vi "Main.vi"(11 "Module Admin":refnum<class "Delacor_lib_QMH_Module Admin.lvclass">) -> ()   [LabVIEW 2024, in "UI Module Template.lvlib"]
doc: "This template is based off of the Queued Message Handler design pattern and the Queued Message Handler project template that ships with LabVIEW.\n\nThe main difference is that the queue is private to this module and communication between modules is performed via Broadcast and Request events.\n\nRequest events are wrapped in public API methods and are handled in the Event Handling Loop (EHL) of this VI. Any module can register for Broadcast events sent by this module. The EHL generates messages based on user interface actions.\n\nThe Message Handling Loop (MHL) processes messages generated by the EHL, or by other messages. The messages are string values, so new messages can be added easily to the Message Cases case structure in the MHL. Each message cluster can also provide an optional value for Message Data, which is a variant that can be converted to whatever message-specific data is required.\n_____\nBased on DQMH Project Template 7.0.1.1316."
uses:
  UI Module Template.lvlib
  <vilib>/Delacor/Delacor QMH/Libraries/Module Admin_class/Delacor_lib_QMH_Module Admin.lvclass
  Module Data--cluster.ctl
  Config.ctl
  <vilib>/Delacor/Delacor QMH/Libraries/Message Queue_class/Delacor_lib_QMH_Message Queue.lvclass/Delacor_lib_QMH_Message Queue.ctl
  Stop Argument--cluster.ctl
  <vilib>/Delacor/Delacor QMH/Libraries/Module Admin_class/Delacor_lib_QMH_Module Admin.lvclass/Delacor_lib_QMH_Module Admin.ctl
  Get UI Reference Argument--cluster.ctl
  Get UI Reference (Reply Payload)--cluster.ctl
  Inserted Into Subpanel Argument--cluster.ctl
  Set Config (String) Argument--cluster.ctl
  Set Config Argument--cluster.ctl
  Get config Argument--cluster.ctl
  Get config (Reply Payload)--cluster.ctl
  Get Config (String) Argument--cluster.ctl
  Get Config (String) (Reply Payload)--cluster.ctl
  Generate Dummy Data Argument--cluster.ctl
  <vilib>/Delacor/Delacor QMH/Libraries/Message Queue_class/Delacor_lib_QMH_Enqueue Message (Single).vi
  <vilib>/Delacor/Delacor QMH/Libraries/Module Admin_class/Delacor_lib_QMH_Get External Launch.vi
  <vilib>/Delacor/Delacor QMH/Libraries/Message Queue_class/Delacor_lib_QMH_Message Queue.lvclass
  <userlib>/_OpenG.lib/appcontrol/appcontrol.llb/openg_application_control.lvlib
panel:
  out "Title":string
  out "error out":errorcluster
  out "Status":string
  in  "Simulate MHL Error":bool
  in  "Simulate EHL Error":bool
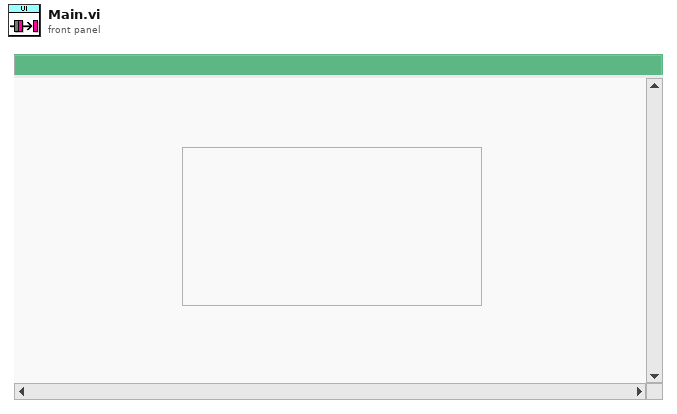
[diagram p1: front panel]
types:
  T1 = typedef "UI Module Template.lvlib/Request Events--cluster.ctl" = cluster{"Stop Module":refnum<user-event>, "Show Panel":refnum<user-event>, "Hide Panel":refnum<user-event>, "Get Module Execution Status":refnum<user-event>, "Show Diagram":refnum<user-event>, "Get UI Reference":refnum<user-event>, "Inserted Into Subpanel":refnum<user-event>, "Set Config (String)":refnum<user-event>, "Set Config":refnum<user-event>, "Get config":refnum<user-event>, "Get Config (String)":refnum<user-event>, "Private":cluster{"Generate Dummy Data":refnum<user-event>}}
  T2 = typedef "UI Module Template.lvlib/Module Data--cluster.ctl" = cluster{"Status":string, "Config":T3}
  T3 = typedef "UI Module Template.lvlib/Config.ctl" = cluster{"<ReplaceMe>":bool}
  T4 = enum32{"invalid lock state", "Not Locked", "Locked (No Password)", "Password-protected"}
  T5 = typedef "UI Module Template.lvlib/Stop Argument--cluster.ctl" = cluster{"Origin":string, "Exit via Stop Module Req?":bool, "Wait for Module to stop?":bool}
  T6 = typedef "UI Module Template.lvlib/Get UI Reference Argument--cluster.ctl" = cluster{"Wait Notifier":refnum<notifier>, "wait for reply":bool}
  T7 = typedef "UI Module Template.lvlib/Inserted Into Subpanel Argument--cluster.ctl" = cluster{"Boolean":bool}
  T8 = typedef "UI Module Template.lvlib/Set Config (String) Argument--cluster.ctl" = cluster{"XML-String":string}
  T9 = typedef "UI Module Template.lvlib/Set Config Argument--cluster.ctl" = cluster{"Config":T3}
  T10 = typedef "UI Module Template.lvlib/Get config Argument--cluster.ctl" = cluster{"Wait Notifier":refnum<notifier>, "wait for reply":bool}
  T11 = typedef "UI Module Template.lvlib/Get Config (String) Argument--cluster.ctl" = cluster{"Wait Notifier":refnum<notifier>, "wait for reply":bool}
  T12 = typedef "UI Module Template.lvlib/Generate Dummy Data Argument--cluster.ctl" = cluster{"Boolean":bool}
  T13 = enum32{"Invalid", "Standard", "Closed", "Hidden", "Minimized", "Maximized"}
  T14 = typedef "UI Module Template.lvlib/Get UI Reference (Reply Payload)--cluster.ctl" = cluster{"UI VI Refnum":refnum<vi>, "error":errorcluster}
  T15 = typedef "UI Module Template.lvlib/Get config (Reply Payload)--cluster.ctl" = cluster{"Config":T3, "error":errorcluster}
  T16 = typedef "UI Module Template.lvlib/Get Config (String) (Reply Payload)--cluster.ctl" = cluster{"Config XML String":string, "error":errorcluster}
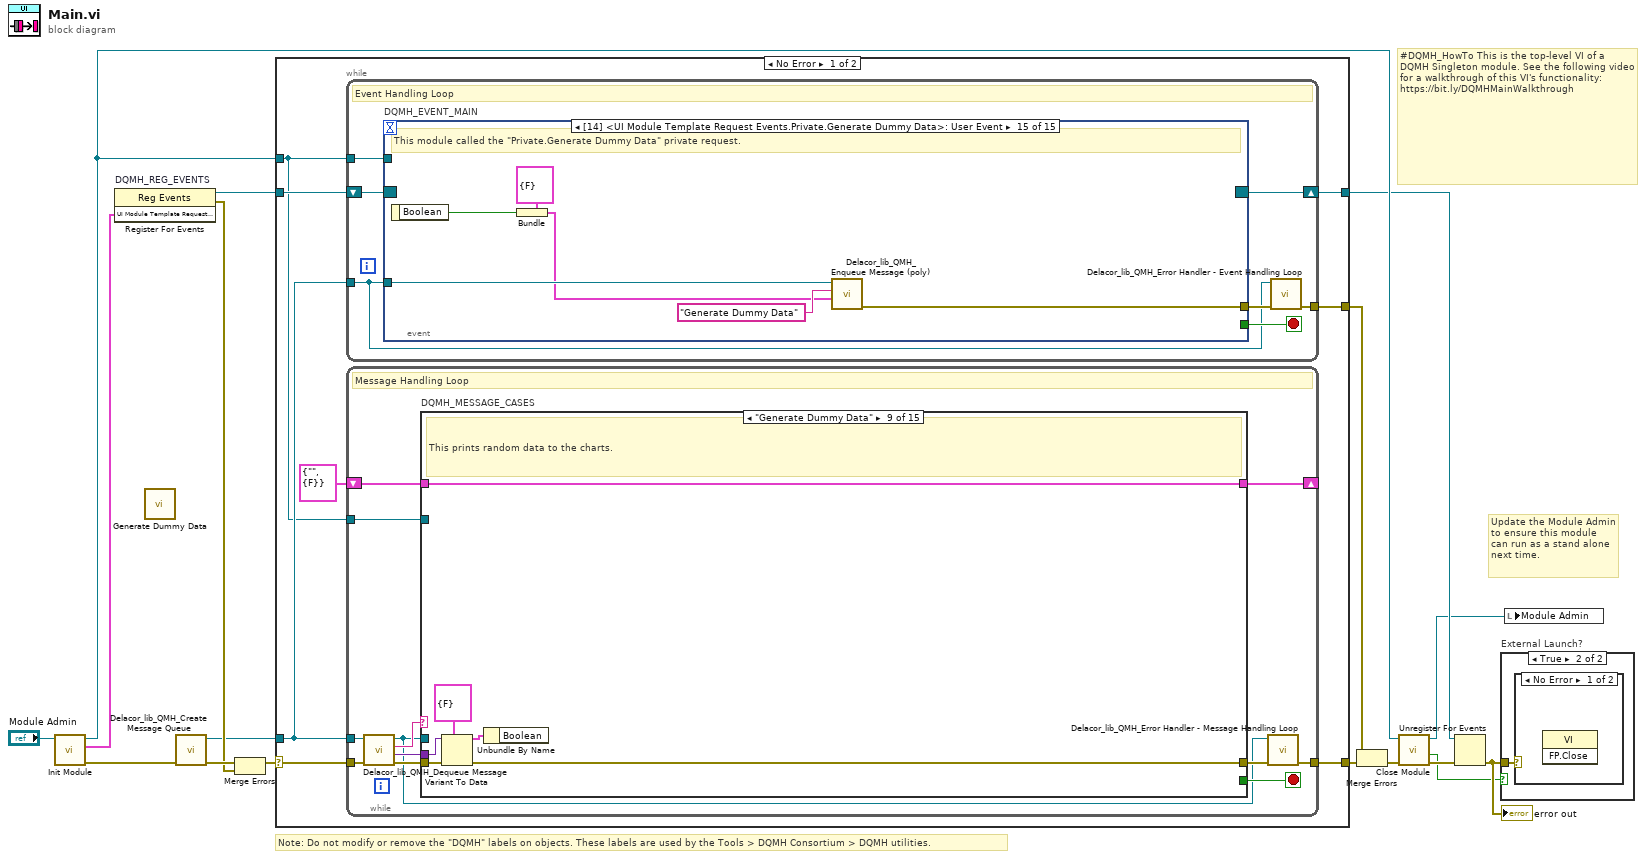
[diagram p0: block diagram]
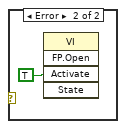
[diagram p3: hidden frame]
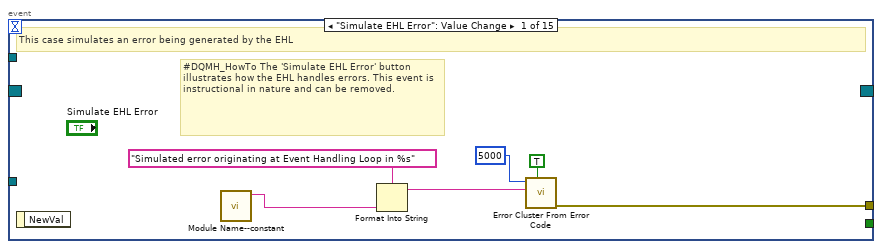
[diagram p4: hidden frame]
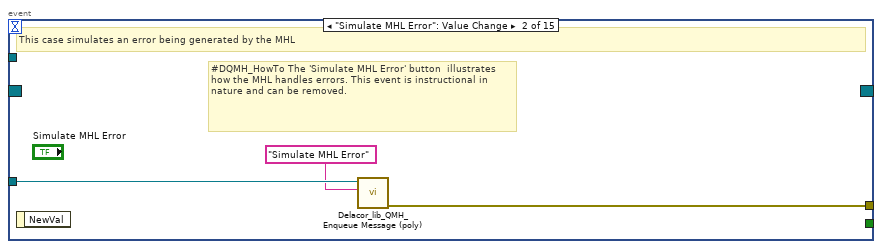
[diagram p5: hidden frame]
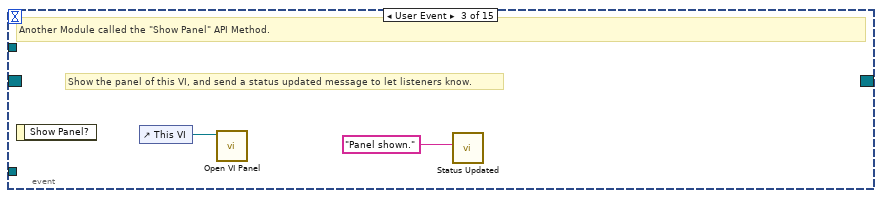
[diagram p6: hidden frame]
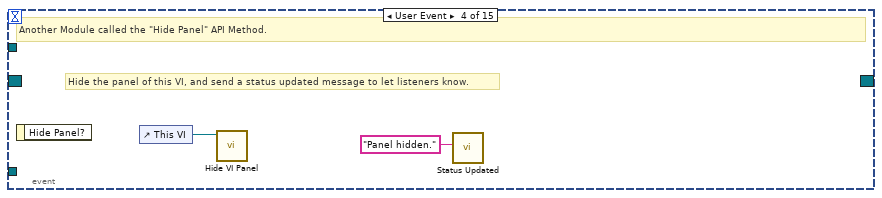
[diagram p7: hidden frame]
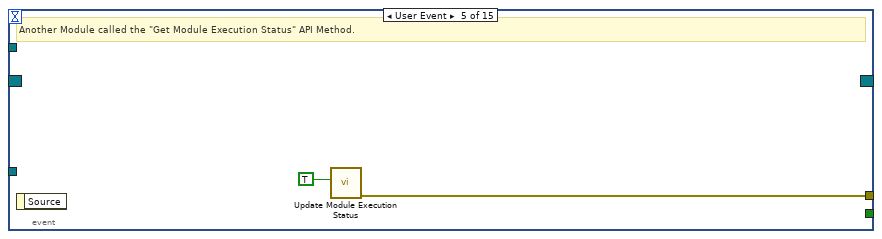
[diagram p8: hidden frame]
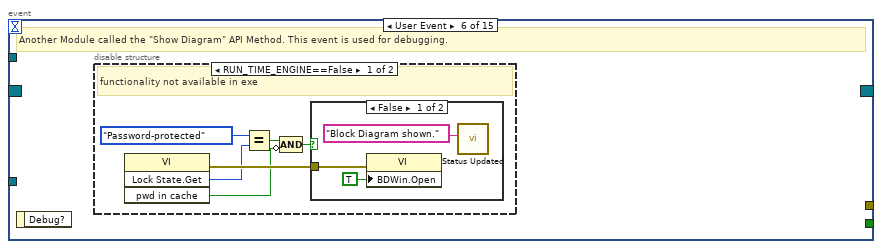
[diagram p9: hidden frame]
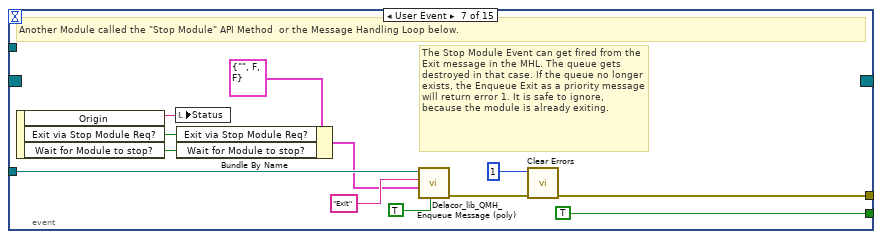
[diagram p12: hidden frame]
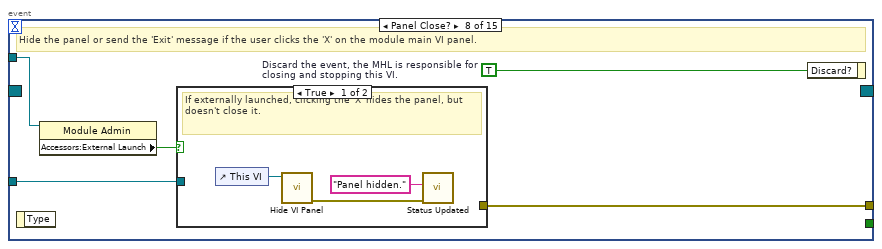
[diagram p13: hidden frame]
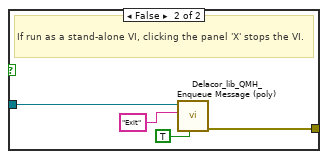
[diagram p14: hidden frame]
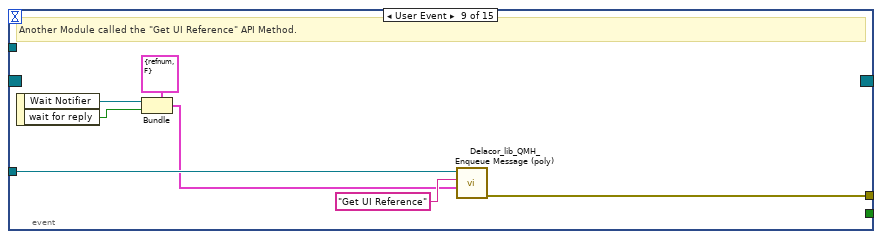
[diagram p15: hidden frame]
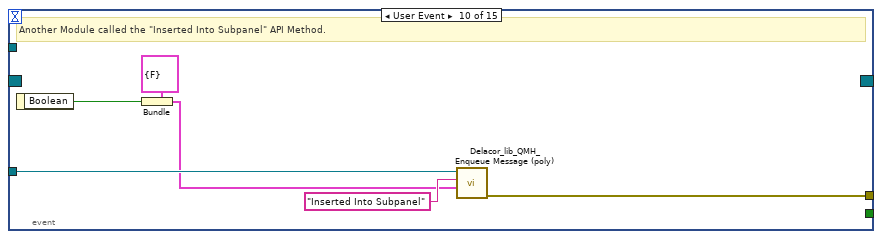
[diagram p16: hidden frame]
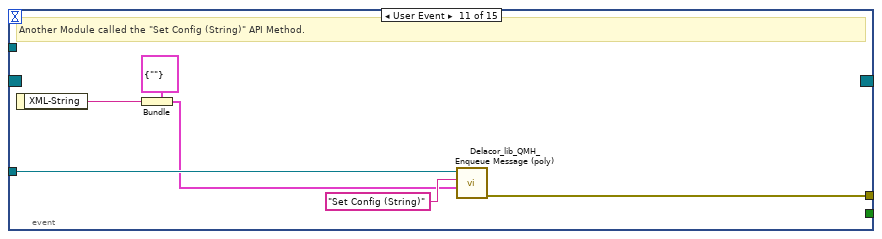
[diagram p17: hidden frame]
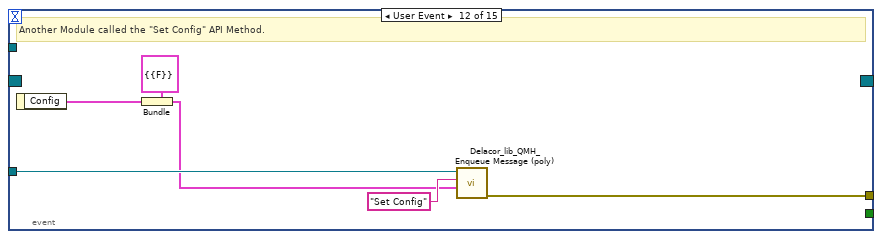
[diagram p18: hidden frame]
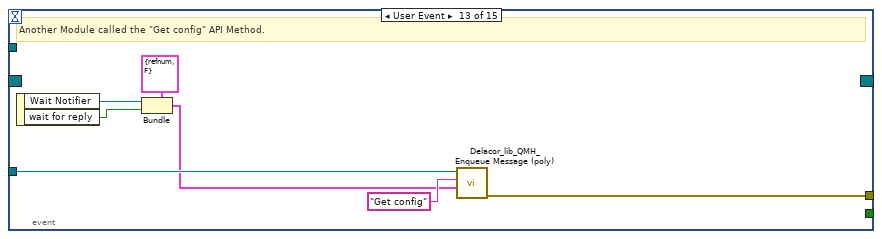
[diagram p19: hidden frame]
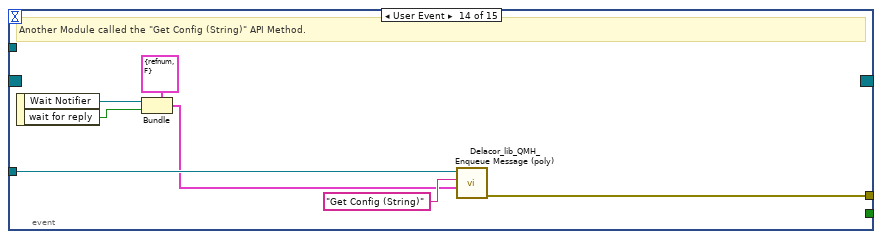
[diagram p20: hidden frame]
diagram:
  # "#DQMH_HowTo This is the top-level VI of a DQMH Singleton module. See the following video for a walkthrough of this VI's functionality: https://bit.ly/DQMHMainWalkthrough"
  # "Note: Do not modify or remove the \"DQMH\" labels on objects. These labels are used by the Tools > DQMH Consortium > DQMH utilities."
  # "Update the Module Admin to ensure this module can run as a stand alone next time."
  n1 = call "Init Module.vi"("Singleton Module Admin in"="Module Admin") -> ("error out"=w16:errorcluster, "UI Module Template Request Events"=w5:T1, "Singleton Module Admin out"=w8:refnum<class "Delacor_lib_QMH_Module Admin.lvclass">)  [unwired: 8 in]
  n2 = register-events "DQMH_REG_EVENTS"(w5) -> (reference out=w6:refnum<event-registration>, error out=w9:errorcluster)  [unwired: 2 in]
  n3 = call "Generate Dummy Data.vi"() -> ()  [unwired: 11 in, 1 out]
  n4 = call <vilib>:"Delacor_lib_QMH_Create Message Queue.vi"("error in"=w16) -> ("error out"=w11:errorcluster, "Message Queue"=w4:refnum<class "Delacor_lib_QMH_Message Queue.lvclass">)  [unwired: 9 in]
  n5 = Merge Errors(w11, w9) -> (w10:errorcluster)
  n6 = case shown="No Error" w10 {
    selector: w10 -> [w23 w290]
    tunnel: [w25 w289] -> w17
    tunnel: [w22 w288] -> w7
    tunnel: w6 -> [w20 w288]
    tunnel: w4 -> [w19 w283]
    tunnel: [w24 _] -> w14
    tunnel: w8 -> [w18 w284]
    frame No Error {
      n7 = while {
        tunnel: w19 -> [w26]
        shift-right: [w29] -> w22
        shift-left: w20 -> [w30]
        tunnel: [w31] -> w24
        tunnel: w18 -> [w27]
        stop <- w28 stop-if-true
        # "Event Handling Loop"
        n8 = event "DQMH_EVENT_MAIN" shown="[14] <UI Module Template Request Events.Private.Generate Dummy Data>: User Event" {
          selector: w30 -> [_ _ _ _ _ _ _ _ _ _ _ _ _ _ _]
          dyn-events: [_ _ _ _ _ _ _ _ _ _ _ _ _ _ _] -> w29
          timeout: _ -> [_ _ _ _ _ _ _ _ _ _ _ _ _ _ _]
          tunnel: [_ _ _ _ _ _ TRUE ("Discard?") _ _ _ _ _ _ _ _] -> w28
          tunnel: w26 -> [_ w40 _ _ _ _ w64 w71 w87 w93 w99 w105 w112 w119 w125]
          tunnel: [w38 w41 _ _ w47 _ w67 w73 w81 w88 w94 w100 w106 w113 w120] -> w32
          tunnel: w27 -> [_ _ _ _ _ _ _ w70 _ _ _ _ _ _ _]
          event "Simulate EHL Error": Value Change {
            # "#DQMH_HowTo The 'Simulate EHL Error' button  illustrates how the EHL handles errors. This event is instructional in nature and can be removed."
            # "This case simulates an error being generated by the EHL"
            n9 = event-data() -> ()  [unwired: 1 in, 1 out]
            n10 = call "Module Name--constant.vi"() -> ("Module Name"=w35:string)  [unwired: 11 in]
            n11 = Format Into String(format string="Simulated error originating at Event Handling Loop in %s", w35) -> (resulting string=w36:string)  [unwired: 2 in, 1 out]
            n12 = call <vilib>:"Error Cluster From Error Code.vi"("show call chain? (False)"=TRUE, "error message (\"\")"=w36, "error code (0)"=5000) -> ("error out"=w38:errorcluster)  [unwired: 6 in]
          }
          event "Simulate MHL Error": Value Change {
            # "#DQMH_HowTo The 'Simulate MHL Error' button  illustrates how the MHL handles errors. This event is instructional in nature and can be removed."
            # "This case simulates an error being generated by the MHL"
            n13 = event-data() -> ()  [unwired: 1 in, 1 out]
            n14 = call-poly <vilib>:"Delacor_lib_QMH_Enqueue Message (poly).vi"("Message"="Simulate MHL Error", "Message Queue in"=w40) -> ("error out"=w41:errorcluster)  [unwired: 8 in, 1 out]
          }
          event User Event {
            # "Show the panel of this VI, and send a status updated message to let listeners know."
            # "Another Module called the \"Show Panel\" API Method."
            n15 = event-data() -> ()  [unwired: 1 in, 1 out]
            n16 = control-ref of="This VI"() -> (w43:refnum<vi>)
            n17 = call "Open VI Panel.vi"("VI"=w43) -> ()  [unwired: 10 in, 1 out]
            n18 = call "Status Updated.vi"("Status"="Panel shown." ("format string")) -> ()  [unwired: 10 in, 1 out]
          }
          event User Event {
            # "Hide the panel of this VI, and send a status updated message to let listeners know."
            # "Another Module called the \"Hide Panel\" API Method."
            n19 = event-data() -> ()  [unwired: 1 in, 1 out]
            n20 = control-ref of="This VI"() -> (w45:refnum<vi>)
            n21 = call "Hide VI Panel.vi"("VI"=w45) -> ()  [unwired: 10 in, 1 out]
            n22 = call "Status Updated.vi"("Status"="Panel hidden." ("format string")) -> ()  [unwired: 10 in, 1 out]
          }
          event User Event {
            # "Another Module called the \"Get Module Execution Status\" API Method."
            n23 = event-data() -> ()  [unwired: 1 in, 1 out]
            n24 = call "Update Module Execution Status.vi"("Running?"=TRUE) -> ("error out"=w47:errorcluster)  [unwired: 10 in]
          }
          event User Event {
            # "Another Module called the \"Show Diagram\" API Method. This event is used for debugging."
            n25 = event-data() -> ()  [unwired: 1 in, 1 out]
            n26 = disable-structure shown="RUN_TIME_ENGINE==False" {
              frame condition #0 (active) {
                # "functionality not available in exe"
                n27 = invoke on="Invoke Node" class="VI" method="Lock State.Get"() -> (error out=w53:errorcluster, "Get Lock State"=w52:T4, "pwd in cache"=w49:bool)  [unwired: 4 in, 1 out]
                n28 = Equal?(x=T4."Password-protected", y=w52) -> (x = y?=w50:bool)
                n29 = Compound Arithmetic op=AND(w50, invert w49) -> (w48:bool)
                n30 = case shown="False" w48 {
                  tunnel: w53 -> [w56 _]
                  frame False {
                    n31 = property on="Property Node" class="VI"(error in=w56, "BDWin.Open"=TRUE ("Block Diagram Window:Open")) -> ()  [unwired: 1 in, 2 out]
                    n32 = call "Status Updated.vi"("Status"="Block Diagram shown." ("format string")) -> ()  [unwired: 10 in, 1 out]
                  }
                  frame True {
                    # "Password-protected VI, and the password is not in the cache. Do not show the diagram."
                  }
                }
              }
              frame condition #1 {
              }
            }
          }
          event User Event {
            # "The Stop Module Event can get fired from the Exit message in the MHL. The queue gets destroyed in that case. If the queue no longer exists, the Enqueue Exit as a priority message will return error 1. It is safe to ignore, because the module is already exiting."
            # "Another Module called the \"Stop Module\" API Method  or the Message Handling Loop below."
            n33 = event-data() -> ("Origin"=w63:string, "Exit via Stop Module Req?"=w59:bool, "Wait for Module to stop?"=w58:bool)  [unwired: 1 in]
            n34 = local write "Status"(w63) -> ()
            n35 = Bundle By Name(cluster=T5 {"Origin"="", "Exit via Stop Module Req?"=FALSE, "Wait for Module to stop?"=FALSE} ("Stop Argument"), "Exit via Stop Module Req?"=w59, "Wait for Module to stop?"=w58) -> (w57:T5)
            n36 = call-poly <vilib>:"Delacor_lib_QMH_Enqueue Message (poly).vi"("Priority Message? (F)"=TRUE, "Message Data"=w57, "Message"="Exit", "Message Queue in"=w64) -> ("error out"=w68:errorcluster)  [unwired: 6 in, 1 out]
            n37 = call <vilib>:"Clear Errors.vi"("error in (no error)"=w68, "specific error code to clear (0: all)"=1) -> ("error out"=w67:errorcluster)  [unwired: 4 in, 1 out]
          }
          event Panel Close? {
            w72 = TRUE  # Discard the event, the MHL is responsible for closing and stopping this VI.
            # "Hide the panel or send the 'Exit' message if the user clicks the 'X' on the module main VI panel."
            n38 = event-data() -> ()  [unwired: 1 in, 1 out]
            n39 = property on="Property Node" class="Module Admin"(reference=w70) -> ("Accessors:External Launch"=w69:bool)  [unwired: 1 in, 2 out]
            n40 = case shown="True" w69 {
              tunnel: w71 -> [_ w79]
              tunnel: [_ w80] -> w73
              frame True {
                # "If externally launched, clicking the 'X' hides the panel, but doesn't close it."
                n41 = control-ref of="This VI"() -> (w76:refnum<vi>)
                n42 = call "Hide VI Panel.vi"("VI"=w76) -> ("error out"=w74:errorcluster)  [unwired: 10 in]
                n43 = call "Status Updated.vi"("error in"=w74, "Status"="Panel hidden." ("format string")) -> ()  [unwired: 9 in, 1 out]
              }
              frame False {
                # "If run as a stand-alone VI, clicking the panel 'X' stops the VI."
                n44 = call-poly <vilib>:"Delacor_lib_QMH_Enqueue Message (poly).vi"("Priority Message? (F)"=TRUE, "Message"="Exit", "Message Queue in"=w79) -> ("error out"=w80:errorcluster)  [unwired: 7 in, 1 out]
              }
            }
            n45 = event-data ("Event Filter Node")("Discard?"=w72) -> ()  [unwired: 1 in, 1 out]
          }
          event User Event {
            # "Another Module called the \"Get UI Reference\" API Method."
            n46 = event-data() -> ("Wait Notifier"=w83:refnum<notifier>, "wait for reply"=w82:bool)  [unwired: 1 in]
            n47 = Bundle(cluster=T6 {"Wait Notifier"=refnum, "wait for reply"=FALSE} ("Get UI Reference Argument"), "Wait Notifier"=w83, "wait for reply"=w82) -> (w84:T6)
            n48 = call-poly <vilib>:"Delacor_lib_QMH_Enqueue Message (poly).vi"("Message Data"=w84, "Message"="Get UI Reference", "Message Queue in"=w87) -> ("error out"=w81:errorcluster)  [unwired: 7 in, 1 out]
          }
          event User Event {
            # "Another Module called the \"Inserted Into Subpanel\" API Method."
            n49 = event-data() -> ("Boolean"=w89:bool)  [unwired: 1 in]
            n50 = Bundle(cluster=T7 {"Boolean"=FALSE} ("Inserted Into Subpanel Argument"), "Boolean"=w89) -> (w90:T7)
            n51 = call-poly <vilib>:"Delacor_lib_QMH_Enqueue Message (poly).vi"("Message Data"=w90, "Message"="Inserted Into Subpanel", "Message Queue in"=w93) -> ("error out"=w88:errorcluster)  [unwired: 7 in, 1 out]
          }
          event User Event {
            # "Another Module called the \"Set Config (String)\" API Method."
            n52 = event-data() -> ("XML-String"=w95:string)  [unwired: 1 in]
            n53 = Bundle(cluster=T8 {"XML-String"=""} ("Set Config (String) Argument"), "XML-String"=w95) -> (w96:T8)
            n54 = call-poly <vilib>:"Delacor_lib_QMH_Enqueue Message (poly).vi"("Message Data"=w96, "Message"="Set Config (String)", "Message Queue in"=w99) -> ("error out"=w94:errorcluster)  [unwired: 7 in, 1 out]
          }
          event User Event {
            # "Another Module called the \"Set Config\" API Method."
            n55 = event-data() -> ("Config"=w101:T3)  [unwired: 1 in]
            n56 = Bundle(cluster=T9 {"Config"={"<ReplaceMe>"=FALSE}} ("Set Config Argument"), "Config"=w101) -> (w102:T9)
            n57 = call-poly <vilib>:"Delacor_lib_QMH_Enqueue Message (poly).vi"("Message Data"=w102, "Message"="Set Config", "Message Queue in"=w105) -> ("error out"=w100:errorcluster)  [unwired: 7 in, 1 out]
          }
          event User Event {
            # "Another Module called the \"Get config\" API Method."
            n58 = event-data() -> ("Wait Notifier"=w108:refnum<notifier>, "wait for reply"=w107:bool)  [unwired: 1 in]
            n59 = Bundle(cluster=T10 {"Wait Notifier"=refnum, "wait for reply"=FALSE} ("Get config Argument"), "Wait Notifier"=w108, "wait for reply"=w107) -> (w109:T10)
            n60 = call-poly <vilib>:"Delacor_lib_QMH_Enqueue Message (poly).vi"("Message Data"=w109, "Message"="Get config", "Message Queue in"=w112) -> ("error out"=w106:errorcluster)  [unwired: 7 in, 1 out]
          }
          event User Event {
            # "Another Module called the \"Get Config (String)\" API Method."
            n61 = event-data() -> ("Wait Notifier"=w115:refnum<notifier>, "wait for reply"=w114:bool)  [unwired: 1 in]
            n62 = Bundle(cluster=T11 {"Wait Notifier"=refnum, "wait for reply"=FALSE} ("Get Config (String) Argument"), "Wait Notifier"=w115, "wait for reply"=w114) -> (w116:T11)
            n63 = call-poly <vilib>:"Delacor_lib_QMH_Enqueue Message (poly).vi"("Message Data"=w116, "Message"="Get Config (String)", "Message Queue in"=w119) -> ("error out"=w113:errorcluster)  [unwired: 7 in, 1 out]
          }
          event User Event {
            # "This module called the \"Private.Generate Dummy Data\" private request."
            n64 = event-data() -> ("Boolean"=w121:bool)  [unwired: 1 in]
            n65 = Bundle(cluster=T12 {"Boolean"=FALSE} ("Generate Dummy Data Argument"), "Boolean"=w121) -> (w122:T12)
            n66 = call-poly <vilib>:"Delacor_lib_QMH_Enqueue Message (poly).vi"("Message Data"=w122, "Message"="Generate Dummy Data", "Message Queue in"=w125) -> ("error out"=w120:errorcluster)  [unwired: 7 in, 1 out]
          }
        }
        n67 = call-dynamic "Delacor_lib_QMH_Error Handler - Event Handling Loop.vi"("error in"=w32, "Message Queue in"=w26) -> ("dup error in"=w31:errorcluster)  [unwired: 8 in, 1 out]
      }
      n68 = while {
        tunnel: w19 -> [w126]
        shift-right: [w134] -> _
        shift-left: T2 {"Status"="", "Config"={"<ReplaceMe>"=FALSE}} ("Data Cluster") -> [w135]
        tunnel: w23 -> [w137]
        tunnel: [w129] -> w25
        tunnel: w18 -> [w130]
        stop <- w133 stop-if-true
        # "Message Handling Loop"
        n69 = call-dynamic "Delacor_lib_QMH_Dequeue Message.vi"("error in"=w137, "Message Queue in"=w126) -> ("error out"=w136:errorcluster, "Message Data"=w131:variant, "Message"=w132:string, "Message Queue out"=w127:refnum<class "Delacor_lib_QMH_Message Queue.lvclass">)  [unwired: 6 in]
        n70 = case "DQMH_MESSAGE_CASES" shown="\"Generate Dummy Data\"" w132 {
          selector: w132 -> [_ _ _ _ _ _ _ _ _ _ _ _ _ _ w278]
          tunnel: w127 -> [_ _ _ _ _ _ _ _ _ _ _ _ w244 w266 _]
          tunnel: w136 -> [w154 w158 w170 w173 w185 w191 w203 w218 w226 w229 w231 w240 w251 w272 w281]
          tunnel: [w152 w158 w160 w173 w179 w189 w194 w209 w224 w228 w231 w239 w247 w267 w282] -> w128
          tunnel: w135 -> [w143 w157 w169 w174 w184 w190 w193 w208 w225 w227 w230 w237 w246 w265 w279]
          tunnel: [w142 w157 w169 w174 w176 w190 w193 w208 w225 w227 w230 w237 w246 w265 w279] -> w134
          tunnel: [_ _ _ _ _ _ _ _ _ _ _ _ _ w264 _] -> w133
          tunnel: w131 -> [_ _ w167 _ w182 w188 w201 w216 w223 _ _ _ w245 w263 _]
          tunnel: w130 -> [w144 _ _ _ _ _ _ _ _ _ _ _ w243 w258 _]
          frame "Initialize" {
            w139 = "Initial Message" ("Initial Message")
            # "#UI_Module Close window instead of\n\"hidden\" to insert into subpanel"
            # "Initialize - Any operation that needs to be done before the module can receive messages. Synchronize Caller Events.vi will inform Start Module.vi that the module has launched and is ready to receive messages. Module Did Init.vi will broadcast that the module initialized."
            n71 = call "Synchronize Caller Events.vi"("error in"=w154, "Singleton Module Admin in"=w144) -> ("error out"=w153:errorcluster, "Singleton Module Admin out"=w140:refnum<class "Delacor_lib_QMH_Module Admin.lvclass">)  [unwired: 8 in]
            n72 = property on="Property Node" class="Module Admin"(reference=w140) -> ("Accessors:External Launch"=w148:bool)  [unwired: 1 in, 2 out]
            n73 = Select(t=T13."Closed" ("State"), s=w148, f=T13."Standard" ("State")) -> (s? t:f=w145:T13)
            n74 = call "Module Name--constant.vi"() -> ("Module Name"=w151:string)  [unwired: 11 in]
            n75 = property on="Property Node" class="VI"("Front Panel.Title"=w151) -> (reference out=w150:refnum<vi>, error out=w156:errorcluster)  [unwired: 2 in]
            n76 = call "Module Name--constant.vi"() -> ("Module Name"=w138:string)  [unwired: 11 in]
            "Title" <- w138
            n77 = invoke on="Invoke Node" class="VI" method="FP.Open"(reference=w150, error in=w156, "State"=w145) -> (reference out=w149:refnum<vi>, error out=w155:errorcluster)  [unwired: 2 in, 3 out]
            n78 = Bundle By Name(cluster=w143, "Status"=w139) -> (w142:T2)
            n79 = call "Module Did Init.vi"("error in"=w153, "Initialized?"=TRUE, "Origin"=w138) -> ("error out"=w152:errorcluster)  [unwired: 8 in]
            n80 = invoke on="Invoke Node" class="VI" method="FP.Center"(reference=w149, error in=w155) -> ()  [unwired: 1 in, 3 out]
            "Status" <- w139
          }
          frame "---Module Specific---" {
            # "Separator -- The following cases handle messages specific to this Module."
          }
          frame "Get UI Reference" {
            # "Returns the VI Reference of the UI of the Module, usually the main.vi. Use this to insert the Module into a sub-panel."
            n81 = Variant To Data(error in=w170, type=T6 {"Wait Notifier"=refnum, "wait for reply"=FALSE} ("Get UI Reference Argument"), Variant=w167) -> (data=w165:T6, error out=w168:errorcluster)
            n82 = Unbundle By Name(w165) -> ("Wait Notifier"=w164:refnum<notifier>, "wait for reply"=w163:bool)
            n83 = call <userlib>:"Current VIs Reference__ogtk.vi"() -> ("Current VI's reference"=w159:refnum<vi>)  [unwired: 5 in]
            n84 = Bundle By Name(cluster=T14 {"UI VI Refnum"=refnum, "error"={"status"=FALSE, "code"=0, "source"=""}} ("Get UI Reference (Reply Payload)"), "UI VI Refnum"=w159) -> (w162:T14)
            n85 = Merge Errors(w168) -> (w160:errorcluster)
            n86 = case "DQMH_FIRE_NOTIFIER" shown="True" w163 {
              tunnel: w164 -> [_ w172]
              tunnel: w162 -> [_ w171]
              frame False {
              }
              frame True {
                n87 = Send Notification(notification=w171, notifier=w172) -> ()  [unwired: 1 in, 2 out]
              }
            }
          }
          frame "Inserted Into Subpanel" {
            # "#UI_Module Update UI when inserted into a subpanel"
            # "This Request is called when the UI VI is inserted into a subpanel."
          }
          frame "Set Config (String)" {
            # "Sets the config data by String of the flattened config.ctl cluster."
            n88 = Variant To Data(error in=w185, type=T8 {"XML-String"=""} ("Set Config (String) Argument"), Variant=w182) -> (data=w180:T8, error out=w183:errorcluster)
            n89 = Unbundle By Name(w180) -> ("XML-String"=w178:string)
            n90 = Unflatten From XML(xml string=w178, type=T3 {"<ReplaceMe>"=FALSE} ("Config"), error in (no error)=w183) -> (value=w175:T3, error out=w179:errorcluster)
            n91 = Bundle By Name(cluster=w184, "Config"=w175) -> (w176:T2)
          }
          frame "Set Config" {
            # "#CodeNeeded\n1. Configure this Message Case for handling the \"Set Config\" message.\n2. Delete or edit this label when done."
            # "Sets the config data for the module."
            n92 = Variant To Data(error in=w191, type=T9 {"Config"={"<ReplaceMe>"=FALSE}} ("Set Config Argument"), Variant=w188) -> (data=w186:T9, error out=w189:errorcluster)
            n93 = Unbundle By Name(w186) -> ()  [unwired: 1 out]
          }
          frame "Get config" {
            # "Returns the modules Config."
            n94 = Variant To Data(error in=w203, type=T10 {"Wait Notifier"=refnum, "wait for reply"=FALSE} ("Get config Argument"), Variant=w201) -> (data=w199:T10, error out=w202:errorcluster)
            n95 = Unbundle By Name(w199) -> ("Wait Notifier"=w198:refnum<notifier>, "wait for reply"=w197:bool)
            n96 = Unbundle By Name(w193) -> ("Config"=w192:T3)
            n97 = Bundle By Name(cluster=T15 {"Config"={"<ReplaceMe>"=FALSE}, "error"={"status"=FALSE, "code"=0, "source"=""}} ("Get config (Reply Payload)"), "Config"=w192) -> (w196:T15)
            n98 = Merge Errors(w202) -> (w194:errorcluster)
            n99 = case "DQMH_FIRE_NOTIFIER" shown="True" w197 {
              tunnel: w198 -> [_ w205]
              tunnel: w196 -> [_ w204]
              frame False {
              }
              frame True {
                n100 = Send Notification(notification=w204, notifier=w205) -> ()  [unwired: 1 in, 2 out]
              }
            }
          }
          frame "Get Config (String)" {
            # "Returns the modules config as an xml string."
            n101 = Variant To Data(error in=w218, type=T11 {"Wait Notifier"=refnum, "wait for reply"=FALSE} ("Get Config (String) Argument"), Variant=w216) -> (data=w214:T11, error out=w217:errorcluster)
            n102 = Unbundle By Name(w214) -> ("Wait Notifier"=w213:refnum<notifier>, "wait for reply"=w212:bool)
            n103 = Unbundle By Name(w208) -> ("Config"=w207:T3)
            n104 = Flatten To XML(6:w207) -> (2:w206:string)
            n105 = Bundle By Name(cluster=T16 {"Config XML String"="", "error"={"status"=FALSE, "code"=0, "source"=""}} ("Get Config (String) (Reply Payload)"), "Config XML String"=w206) -> (w211:T16)
            n106 = Merge Errors(w217) -> (w209:errorcluster)
            n107 = case "DQMH_FIRE_NOTIFIER" shown="True" w212 {
              tunnel: w213 -> [_ w220]
              tunnel: w211 -> [_ w219]
              frame False {
              }
              frame True {
                n108 = Send Notification(notification=w219, notifier=w220) -> ()  [unwired: 1 in, 2 out]
              }
            }
          }
          frame "Generate Dummy Data" {
            # "This prints random data to the charts."
            n109 = Variant To Data(error in=w226, type=T12 {"Boolean"=FALSE} ("Generate Dummy Data Argument"), Variant=w223) -> (data=w221:T12, error out=w224:errorcluster)
            n110 = Unbundle By Name(w221) -> ()  [unwired: 1 out]
          }
          frame "---Copy This Frame---" {
            # "Duplicate this frame when creating new messages.  Change this comment in the duplicated frame to describe this message."
            n111 = Merge Errors(w229) -> (w228:errorcluster)
          }
          frame "---Exit and Error Handling---" {
            # "Separator - The following cases handle errors and exit messages."
          }
          frame "Simulate MHL Error" {
            # "#DQMH_HowTo The 'Simulate MHL Error' button  illustrates how the MHL handles errors. This event is instructional in nature and can be removed."
            # "Simulate an error occurring at the MHL"
            n112 = call "Module Name--constant.vi"() -> ("Module Name"=w233:string)  [unwired: 11 in]
            n113 = Format Into String(format string="Simulated error originating at Message Handling Loop in %s", w233) -> (resulting string=w234:string)  [unwired: 2 in, 1 out]
            n114 = call <vilib>:"Error Cluster From Error Code.vi"("show call chain? (False)"=TRUE, "error message (\"\")"=w234, "error code (0)"=5001) -> ("error out"=w238:errorcluster)  [unwired: 6 in]
            n115 = Merge Errors(w240, w238) -> (w239:errorcluster)
          }
          frame "Error" {
            # "Error - Check the error message data and respond accordingly. This message is sent by the \"Error Handler\" VIs at the end of each loop in this application."
            n116 = property on="Property Node" class="Module Admin"(reference=w243) -> ("Accessors:External Launch"=w242:bool)  [unwired: 1 in, 2 out]
            n117 = Variant To Data(error in=w251, type=errorcluster {"status"=FALSE, "code"=0, "source"=""} ("error constant"), Variant=w245) -> (data=w241:errorcluster, error out=w249:errorcluster)
            n118 = local write "error out"(w241) -> ()
            n119 = call "Error Reported.vi"("Error"=w241) -> ()  [unwired: 10 in, 1 out]
            n120 = case shown="False" w242 {
              tunnel: [w256 _] -> w248
              tunnel: w244 -> [w254 _]
              tunnel: w241 -> [w255 _]
              frame False {
                n121 = disable-structure shown="Default" {
                  disable-tunnel: w255 -> [w257 _]
                  frame condition #0 (active) {
                    # "If the module is running standalone, then pop up an error dialog and call the \"Exit\" message."
                    n122 = call <vilib>:"Simple Error Handler.vi"("error in (no error)"=w257) -> ()  [unwired: 4 in, 5 out]
                  }
                  frame condition #1 {
                    # "To prevent the Simple Error Handler VI from being loaded (e.g. when deploying to a Real-Time target), add the Conditional Disable Symbol \"DQMH_Disable_SEH\" to your project and set it to TRUE."
                  }
                }
                n123 = call-poly <vilib>:"Delacor_lib_QMH_Enqueue Message (poly).vi"("Priority Message? (F)"=TRUE, "Message"="Exit", "Message Queue in"=w254) -> ("error out"=w256:errorcluster)  [unwired: 7 in, 1 out]
              }
              frame True {
                # "If the module was launched externally, calling the Error Reported broadcast VI is the only action performed by the \"Error\" message. The module's caller can then process the error appropriately."
              }
            }
            n124 = Merge Errors(w249, w248) -> (w247:errorcluster)
          }
          frame "Exit" {
            w262 = 91  # 91: not all Exit messages will have an argument
            w264 = TRUE  # Stop the VI
            # "Release the message queue reference"
            # "Exit - Exit the application."
            n125 = Variant To Data(error in=w272, type=T5 {"Origin"="", "Exit via Stop Module Req?"=FALSE, "Wait for Module to stop?"=FALSE} ("Stop Argument"), Variant=w263) -> (data=w260:T5, error out=w269:errorcluster)
            n126 = call <vilib>:"Clear Errors.vi"("error in (no error)"=w269, "specific error code to clear (0: all)"=w262) -> ("error out"=w271:errorcluster)  [unwired: 4 in, 1 out]
            n127 = control-ref of="This VI"() -> (w259:refnum<vi>)
            n128 = call-dynamic "Delacor_lib_QMH_Release Message Queue.vi"("error in"=w271, "Message Queue"=w266) -> ("error out"=w270:errorcluster)  [unwired: 9 in]
            n129 = call "Handle Exit.vi"("Stop Argument"=w260, "Admin in"=w258, "VI reference"=w259) -> ("error out"=w268:errorcluster)  [unwired: 7 in, 1 out]
            n130 = Merge Errors(w270, w268) -> (w267:errorcluster)
            n131 = call "Error Reported.vi"("Error"=w267) -> ()  [unwired: 10 in, 1 out]
          }
          frame Default {
            # "'Default' case only runs if there is a message that isn't defined in any of the other cases.  Output a programming error."
            n132 = call "Module Name--constant.vi"() -> ("Module Name"=w277:string)  [unwired: 11 in]
            n133 = Format Into String(format string="The invalid message string \"%s\" was received in the Message Handling Loop for module \"%s\".", w278, w277) -> (resulting string=w273:string)  [unwired: 2 in, 1 out]
            n134 = call <vilib>:"Error Cluster From Error Code.vi"("show call chain? (False)"=TRUE, "error message (\"\")"=w273, "error code (0)"=1) -> ("error out"=w280:errorcluster)  [unwired: 6 in]
            n135 = Merge Errors(w281, w280) -> (w282:errorcluster)
          }
        }
        n136 = call-dynamic "Delacor_lib_QMH_Error Handler - Message Handling Loop.vi"("error in"=w128, "Message Queue in"=w127) -> ("dup error in"=w129:errorcluster)  [unwired: 8 in, 1 out]
      }
    }
    frame Error {
      # "Synchronize Caller Events.vi will inform Start Module.vi that the module has launched and will let the code calling Start Module.vi register for broadcasts and would permit the caller receive the broadcast that an error occurred at launch time."
      n137 = call-dynamic "Delacor_lib_QMH_Release Message Queue.vi"("error in"=w290, "Message Queue"=w283) -> ("error out"=w289:errorcluster)  [unwired: 9 in]
      n138 = call "Synchronize Caller Events.vi"("Singleton Module Admin in"=w284) -> ("error out"=w291:errorcluster)  [unwired: 9 in, 1 out]
      n139 = call "Module Name--constant.vi"() -> ("Module Name"=w287:string)  [unwired: 11 in]
      n140 = Format Into String(format string="An error occurred during initialization. %s is no longer running.", w287) -> (resulting string=w285:string)  [unwired: 2 in, 1 out]
      n141 = Merge Errors(w289, w291) -> (w292:errorcluster)
      n142 = call "Error Reported.vi"("Additional Information"=w285, "Error"=w292) -> ()  [unwired: 9 in, 1 out]
    }
  }
  n143 = Merge Errors(w14, w17) -> (w13:errorcluster)
  n144 = call "Close Module.vi"("error in"=w13, "Module Admin in"=w8) -> ("error out"=w15:errorcluster, "External Launch"=w1:bool, "Module Admin out"=w2:refnum<class "Delacor_lib_QMH_Module Admin.lvclass">)  [unwired: 7 in]
  n145 = Unregister For Events(event registration refnum=w7, error in=w15) -> (error out=w12:errorcluster)
  "error out" <- w12
  n146 = case "External Launch?" shown="True" w1 {
    tunnel: w12 -> [_ w293]
    frame False {
    }
    frame True {
      n147 = case shown="No Error" w293 {
        frame No Error {
          n148 = invoke on="Invoke Node" class="VI" method="FP.Close"() -> ()  [unwired: 3 in, 3 out]
        }
        frame Error {
          n149 = invoke on="Invoke Node" class="VI" method="FP.Open"("Activate"=TRUE ("Activate?")) -> ()  [unwired: 4 in, 5 out]
        }
      }
    }
  }
  n150 = local write "Module Admin"(w2) -> ()
